vi "Tracepoint_CloseStream.vi"(6 "blocks sent":i32, 8 "error in (no error)":errorcluster, 9 "group":string, 10 "stream Id":string, 11 "Qbus in":refnum<class "Qbus.lvclass">) -> (0 "error out":errorcluster)   [LabVIEW 2017, in "FileManager.lvlib"]
uses:
  <vilib>/addons/InsightCM/Devices/Shared/Common/FileManager/FileManager.lvlib
  <vilib>/addons/Qbus/Qbus.lvclass
  <vilib>/addons/TraceLogger/TraceLogger.lvlib
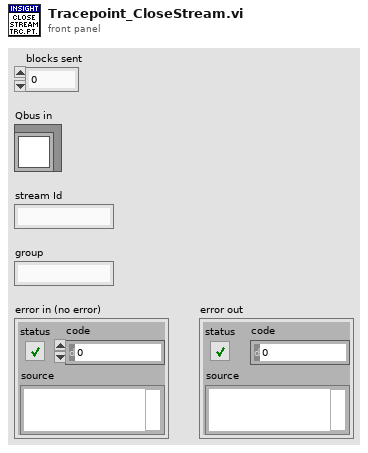
[diagram p1: front panel]
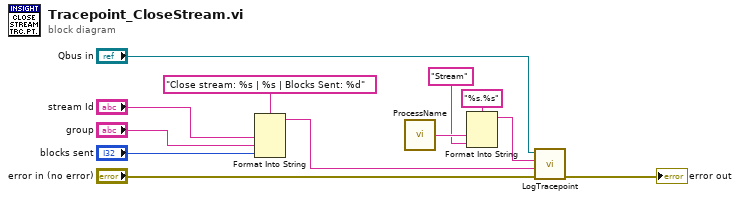
[diagram p0: block diagram]
diagram:
  n1 = Format Into String(format string="Close stream: %s | %s | Blocks Sent: %d", "stream Id", "group", "blocks sent") -> (resulting string=w2:string)  [unwired: 2 in, 1 out]
  n2 = call <vilib>:"ProcessName.vi"() -> ("process name"=w8:string)  [unwired: 5 in]
  n3 = Format Into String(format string="%s.%s", w8, "Stream" ("tracepoint")) -> (resulting string=w5:string)  [unwired: 2 in, 1 out]
  n4 = call <vilib>:"LogTracepoint.vi"("error in (no error)"="error in (no error)", "log string"=w2, "tracepoint"=w5, "qbus in"="Qbus in") -> ("error out"=→"error out":errorcluster)  [unwired: 6 in, 1 out]
